vi "ActuatorCtrl.vi"(7 "P-Gain":dbl, 8 "error in (no error)":errorcluster, 9 "ROSCO Params in":T4, 10 "IO Signals In":T3, 11 "ArrayPairs In":T1={"iStatus"={"Index"=0, "Value"=0.0}, "TIME"={"Index"=1, "Value"=0.0}, "DT"={"Index"=2, "Value"=0.0}, "Blade1PitchPos_rad"={"Index"=3, "Value"=0.0}, "VS_MECHGENPWR"={"Index"=13, "Value"=0.0}, "VS_GENPWR"={"Index"=14, "Value"=0.0}, "GEN_SPEED"={"Index"=19, "Value"=0.0}, "ROTOR_SPEED"={"Index"=20, "Value"=0.0}, "GENTQMEAS"={"Index"=22, "Value"=0.0}, "Y_M"={"Index"=23, "Value"=0.0}, "HORWINDV"={"Index"=26, "Value"=0.0}, "ROOTMOOP1"={"Index"=29, "Value"=0.0}, "ROOTMOOP2"={"Index"=30, "Value"=0.0}, "Blade2PitchPos_rad"={"Index"=32, "Value"=0.0}, "Blade3PitchPos_rad"={"Index"=33, "Value"=0.0}, "ROOTMOOP3"={"Index"=31, "Value"=0.0}, "AVCMSG_SIZE"={"Index"=48, "Value"=0.0}, "INFILE_SIZE "={"Index"=49, "Value"=0.0}, "OUTFILE_SIZE "={"Index"=50, "Value"=0.0}, "FA_ACC"={"Index"=52, "Value"=0.0}, "NUM_BLADES"={"Index"=60, "Value"=0.0}, "BladePitchSetpoint_rad"={"Index"=44, "Value"=0.0}, "TorqueSetpoint_Nm"={"Index"=46, "Value"=0.0}, "OUT_AEROTQ"={"Index"=89, "Value"=0.0}, "Out.RotSpeed "={"Index"=92, "Value"=0.0}, "Out.DEBUG"={"Index"=93, "Value"=0.0}}) -> (0 "error out":errorcluster, 1 "ROSCO Params Out":T4, 2 "IO Signals Out":T3, 3 "ArrayPairs Out":T1={"iStatus"={"Index"=0, "Value"=0.0}, "TIME"={"Index"=1, "Value"=0.0}, "DT"={"Index"=2, "Value"=0.0}, "Blade1PitchPos_rad"={"Index"=3, "Value"=0.0}, "VS_MECHGENPWR"={"Index"=13, "Value"=0.0}, "VS_GENPWR"={"Index"=14, "Value"=0.0}, "GEN_SPEED"={"Index"=19, "Value"=0.0}, "ROTOR_SPEED"={"Index"=20, "Value"=0.0}, "GENTQMEAS"={"Index"=22, "Value"=0.0}, "Y_M"={"Index"=23, "Value"=0.0}, "HORWINDV"={"Index"=26, "Value"=0.0}, "ROOTMOOP1"={"Index"=29, "Value"=0.0}, "ROOTMOOP2"={"Index"=30, "Value"=0.0}, "Blade2PitchPos_rad"={"Index"=32, "Value"=0.0}, "Blade3PitchPos_rad"={"Index"=33, "Value"=0.0}, "ROOTMOOP3"={"Index"=31, "Value"=0.0}, "AVCMSG_SIZE"={"Index"=48, "Value"=0.0}, "INFILE_SIZE "={"Index"=49, "Value"=0.0}, "OUTFILE_SIZE "={"Index"=50, "Value"=0.0}, "FA_ACC"={"Index"=52, "Value"=0.0}, "NUM_BLADES"={"Index"=60, "Value"=0.0}, "BladePitchSetpoint_rad"={"Index"=44, "Value"=0.0}, "TorqueSetpoint_Nm"={"Index"=46, "Value"=0.0}, "OUT_AEROTQ"={"Index"=89, "Value"=0.0}, "Out.RotSpeed "={"Index"=92, "Value"=0.0}, "Out.DEBUG"={"Index"=93, "Value"=0.0}})   [LabVIEW 2018]
uses:
  Clusters/RoscoParams.ctl
  Clusters/IOSignals.ctl
  Clusters/ArrayPairs.ctl
  Clusters/SwapArrayCluster.ctl
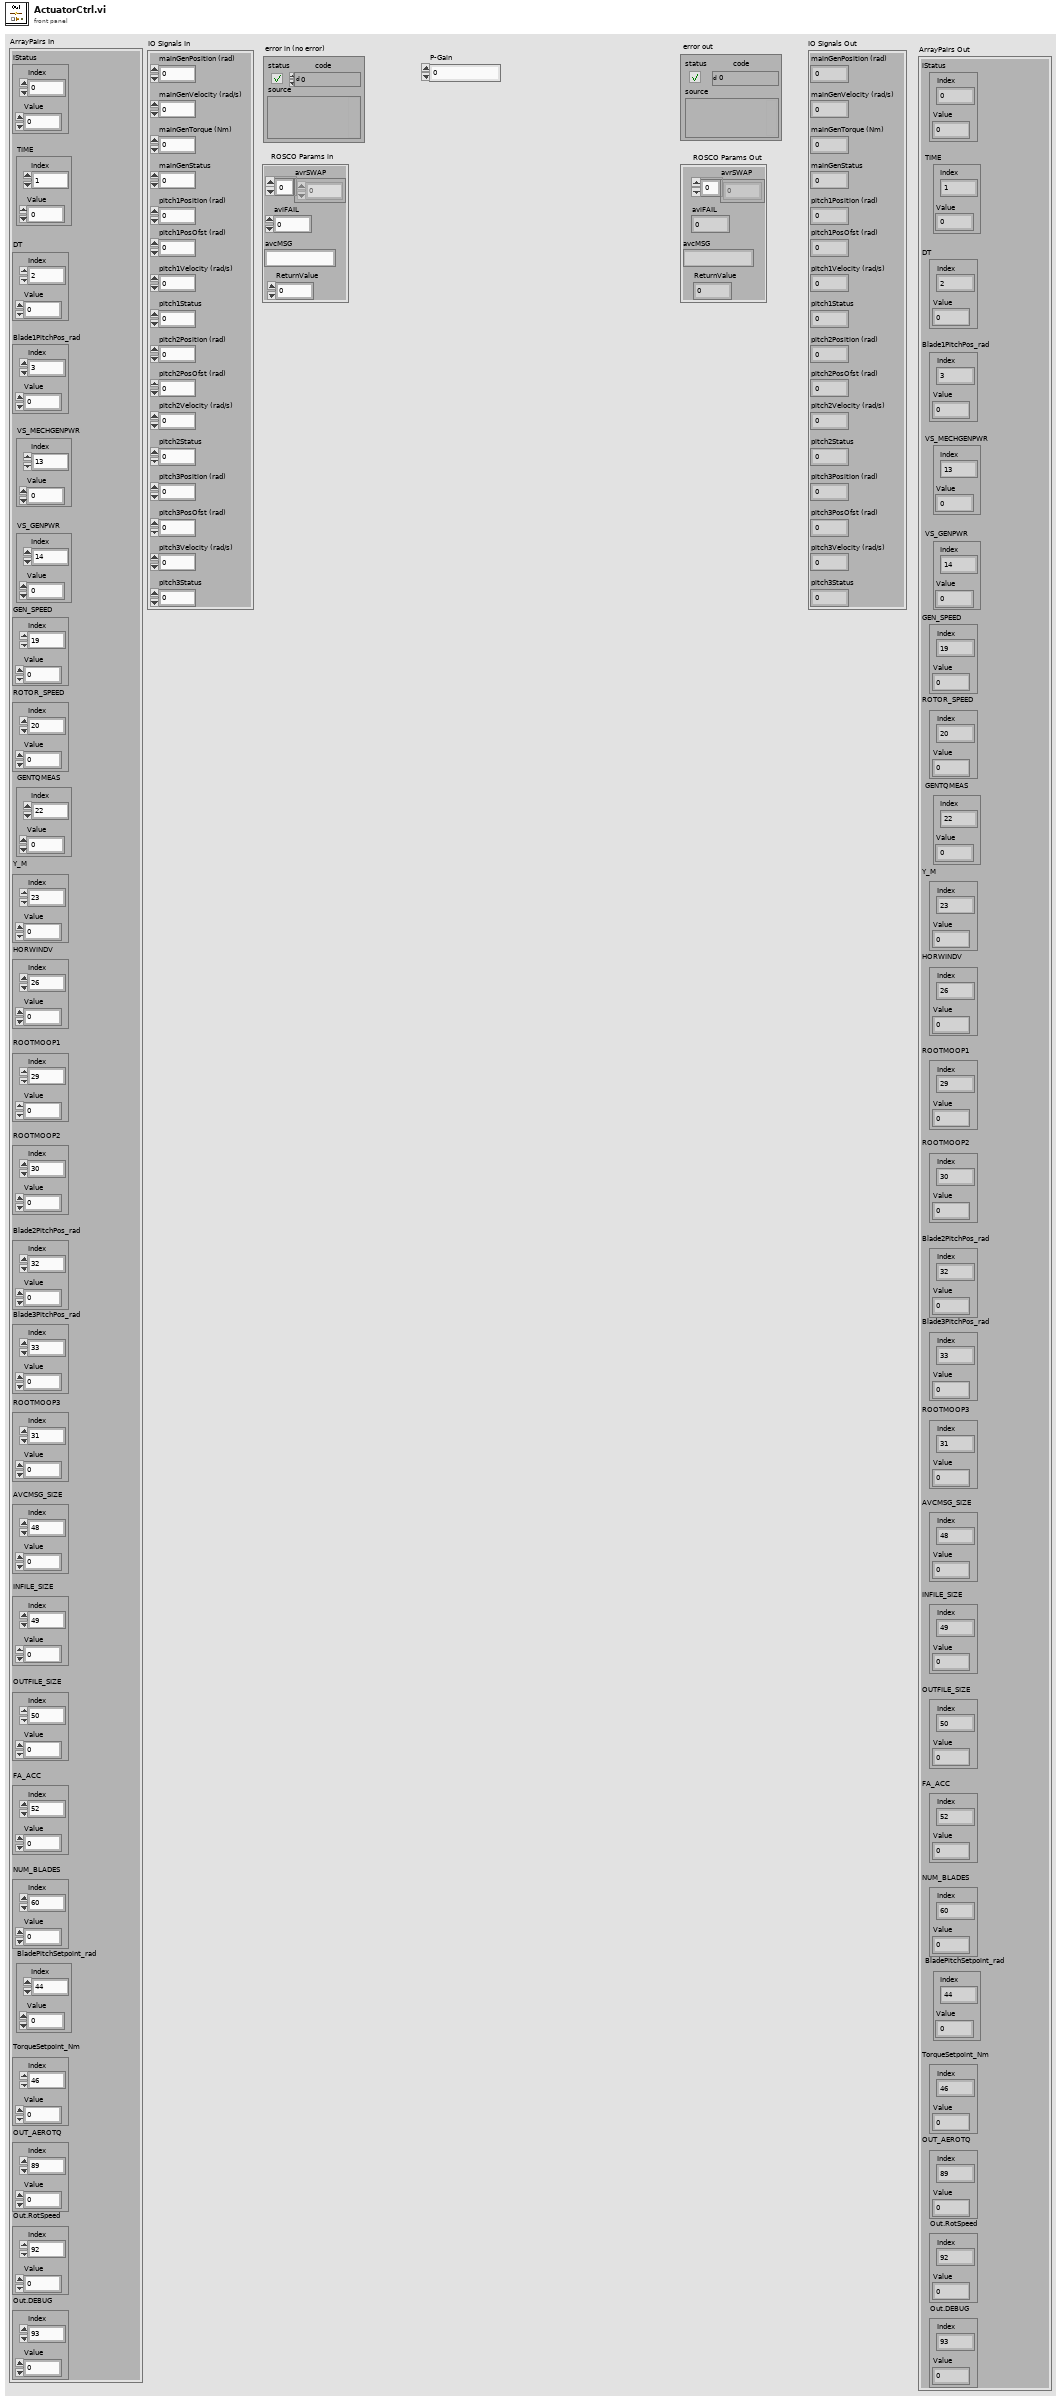
[diagram p1: front panel]
types:
  T1 = typedef "ArrayPairs.ctl" = cluster{"iStatus":T2, "TIME":T2, "DT":T2, "Blade1PitchPos_rad":T2, "VS_MECHGENPWR":T2, "VS_GENPWR":T2, "GEN_SPEED":T2, "ROTOR_SPEED":T2, "GENTQMEAS":T2, "Y_M":T2, "HORWINDV":T2, "ROOTMOOP1":T2, "ROOTMOOP2":T2, "Blade2PitchPos_rad":T2, "Blade3PitchPos_rad":T2, "ROOTMOOP3":T2, "AVCMSG_SIZE":T2, "INFILE_SIZE ":T2, "OUTFILE_SIZE ":T2, "FA_ACC":T2, "NUM_BLADES":T2, "BladePitchSetpoint_rad":T2, "TorqueSetpoint_Nm":T2, "OUT_AEROTQ":T2, "Out.RotSpeed ":T2, "Out.DEBUG":T2}
  T2 = typedef "SwapArrayCluster.ctl" = cluster{"Index":i32, "Value":dbl}
  T3 = typedef "IOSignals.ctl" = cluster{"mainGenPosition (rad)":dbl, "mainGenTorque (Nm)":dbl, "mainGenVelocity (rad/s)":dbl, "mainGenStatus":u16, "pitch1Position (rad)":dbl, "pitch1Velocity (rad/s)":dbl, "pitch1Status":u16, "pitch2Position (rad)":dbl, "pitch2Velocity (rad/s)":dbl, "pitch2Status":u16, "pitch3Position (rad)":dbl, "pitch3Velocity (rad/s)":dbl, "pitch3Status":u16, "pitch1PosOfst (rad)":dbl, "pitch2PosOfst (rad)":dbl, "pitch3PosOfst (rad)":dbl}
  T4 = typedef "RoscoParams.ctl" = cluster{"avrSWAP":sgl[], "aviFAIL":i32, "avcMSG":string, "ReturnValue":i32}
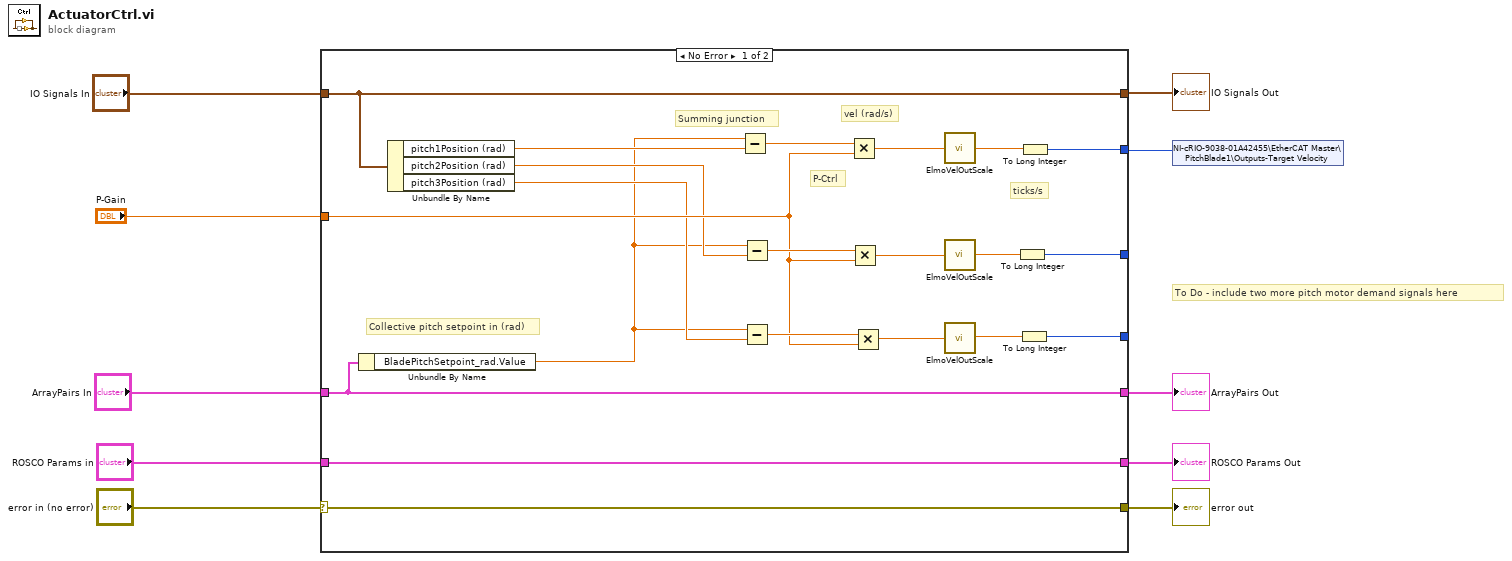
[diagram p0: block diagram]
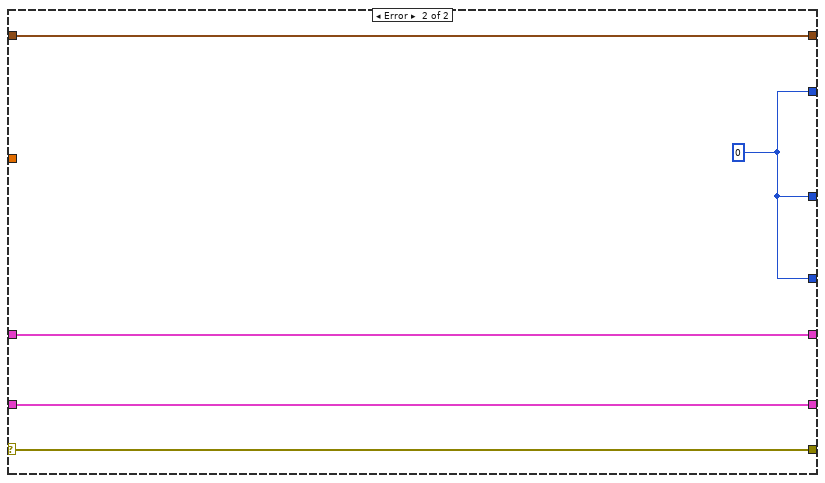
[diagram p2: hidden frame]
diagram:
  # "To Do - include two more pitch motor demand signals here"
  n1 = case shown="No Error" "error in (no error)" {
    selector: "error in (no error)" -> [w31 w36]
    tunnel: [w31 w36] -> w9
    tunnel: [w30 w35] -> w7
    tunnel: "ROSCO Params in" -> [w30 w35]
    tunnel: [w29 w34] -> w5
    tunnel: "ArrayPairs In" -> [w29 w34]
    tunnel: [w28 w33] -> w3
    tunnel: "IO Signals In" -> [w28 w33]
    tunnel: [w27 w32] -> w1
    tunnel: "P-Gain" -> [w20 _]
    tunnel: [w12 w32] -> _
    tunnel: [w11 w32] -> _
    frame No Error {
      # "P-Ctrl"
      # "ticks/s"
      # "vel (rad/s)"
      # "Summing junction"
      # "Collective pitch setpoint in (rad)"
      n2 = Unbundle By Name(w29) -> ("BladePitchSetpoint_rad.Value"=w15:dbl)
      n3 = Unbundle By Name(w28) -> ("pitch1Position (rad)"=w25:dbl, "pitch2Position (rad)"=w17:dbl, "pitch3Position (rad)"=w16:dbl)
      n4 = Subtract(x=w15, y=w25) -> (x-y=w26:dbl)
      n5 = Subtract(x=w15, y=w17) -> (x-y=w22:dbl)
      n6 = Subtract(x=w15, y=w16) -> (x-y=w21:dbl)
      n7 = Multiply(x=w26, y=w20) -> (x*y=w24:dbl)
      n8 = Multiply(x=w22, y=w20) -> (x*y=w19:dbl)
      n9 = Multiply(x=w21, y=w20) -> (x*y=w18:dbl)
      n10 = call "ElmoVelOutScale.vi"("vel (rad/s)"=w24) -> ("vel (tick/s)"=w23:dbl)
      n11 = call "ElmoVelOutScale.vi"("vel (rad/s)"=w19) -> ("vel (tick/s)"=w14:dbl)
      n12 = call "ElmoVelOutScale.vi"("vel (rad/s)"=w18) -> ("vel (tick/s)"=w13:dbl)
      n13 = To Long Integer(number=w14) -> (32bit integer=w12:i32)
      n14 = To Long Integer(number=w13) -> (32bit integer=w11:i32)
      n15 = To Long Integer(number=w23) -> (32bit integer=w27:i32)
    }
    frame Error {
      w32 = 0
    }
  }
  "error out" <- w9
  "ROSCO Params Out" <- w7
  "IO Signals Out" <- w3
  "ArrayPairs Out" <- w5
  n16 = shared-variable "NI-cRIO-9038-01A42455\\EtherCAT Master\\PitchBlade1\\Outputs-Target Velocity"(w1) -> ()  [unwired: 1 in, 1 out]
